vi "FPGA_AIWriteScanList.vi"(8 "error in (no error)":errorcluster, 10 "Scan List":u8[](array[numeric]), 11 "AI Reference":T1) -> (0 "error out":errorcluster, 3 "AI Reference":T1)   [LabVIEW 2017]
uses:
  <vilib>/Rock Robotics/SystemInterfaces/AI/FPGA_AIDevRef.ctl
  <vilib>/Rock Robotics/SystemInterfaces/System/FPGA_SystemFPGA Ref Global.vi
  <vilib>/Utility/error.llb/Error Cluster From Error Code.vi
  <vilib>/rvi/errors/niLvFpgaAdjustHostInterfaceError.vi
  <vilib>/rvi/interface/nirviReadWriteControl/nirviReadWriteControl.xnode
  <vilib>/Rock Robotics/SystemInterfaces/System/FPGA_SystemFRC FPGA Ref.ctl
  NiFpgaLv.dll
  <vilib>/rvi/interface/Simulation/niFpgaSimulationCallBeginRW.vi
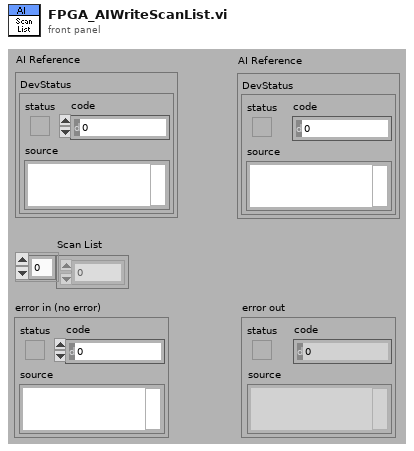
[diagram p1: front panel]
types:
  T1 = typedef "FPGA_AIDevRef.ctl" = cluster{"DevStatus":errorcluster}
  T2 = typedef "FPGA_SystemFRC FPGA Ref.ctl" = refnum<k20>
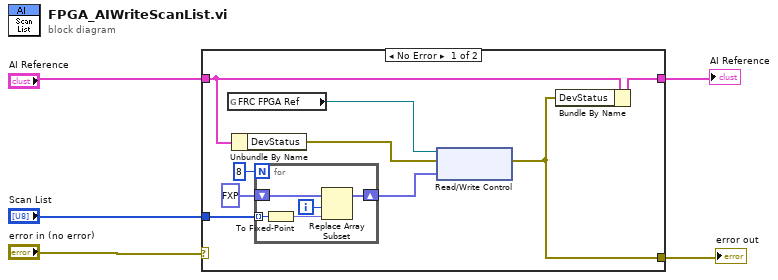
[diagram p0: block diagram]
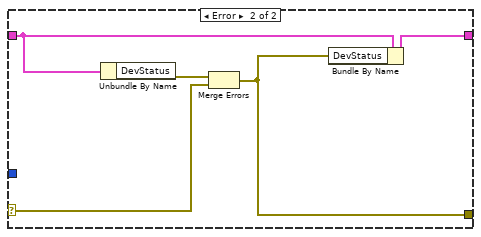
[diagram p2: hidden frame]
diagram:
  n1 = case shown="No Error" "error in (no error)" {
    selector: "error in (no error)" -> [_ w23]
    tunnel: [w6 w20] -> w4
    tunnel: "AI Reference" -> [w14 w22]
    tunnel: [w8 w21] -> w3
    tunnel: "Scan List" -> [w12 _]
    frame No Error {
      n2 = global read "FPGA_SystemFPGA Ref Global.vi" "FRC FPGA Ref"() -> (w7:T2)
      n3 = Unbundle By Name(w14) -> ("DevStatus"=w13:errorcluster)
      n4 = for {
        N: 8 -> [_]
        tunnel: w12 -> [w19] mode=indexing
        shift-right: [w17] -> w11
        shift-left: fxp<+,3,3>[] [0.0, 1.0, 2.0, 3.0, 4.0, 5.0, 6.0, 7.0] ("AI0.ScanList") -> [w18]
        i -> [w15]
        n5 = To Fixed-Point(number=w19) -> (fixed-point=w16:fxp<+,3,3>)  [unwired: 1 out]
        n6 = Replace Array Subset(array=w18, new element=w16, index=w15) -> (w17:fxp<+,3,3>[])
      }
      n7 = xnode "Read/Write Control"("FPGA VI Reference In"=w7, "error in"=w13, "AI.ScanList"=w11) -> ("error out"=w8:errorcluster)  [unwired: 1 out]
      n8 = Bundle By Name(cluster=w14, "DevStatus"=w8) -> (w6:T1)
    }
    frame Error {
      n9 = Unbundle By Name(w22) -> ("DevStatus"=w24:errorcluster)
      n10 = Merge Errors(w24, w23) -> (w21:errorcluster)
      n11 = Bundle By Name(cluster=w22, "DevStatus"=w21) -> (w20:T1)
    }
  }
  "AI Reference" <- w4
  "error out" <- w3
